vi "Circle detection.vi"() -> ()   [LabVIEW 2014]
uses:
  Resources/Global.vi
  <vilib>/vision/NI_Vision_Development_Module.lvlib
panel:
  in  "Circle Index":i32
  out "Number of Matches Returned":i32
  out "error out":errorcluster
  out "Image":T1(plugin-control)
  in  "milliseconds to wait":u32
  out "x-y":u32=19
  # "Do NOT un this VI. Instead run \"AR.Drone MAIN.vi\" and select the name of this VI in the dop-down menu at the Steup tab"
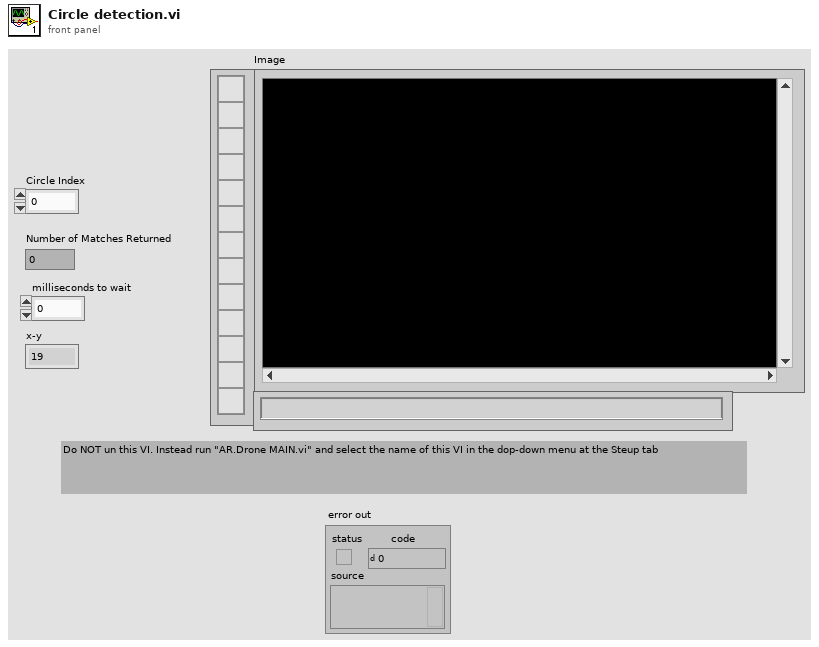
[diagram p1: front panel]
types:
  T1 = typedef "IMAQ Image.ctl" = refnum<image>
  T2 = typedef "Image Type" = u32
  T3 = cluster{"Position":cluster{"X":sgl, "Y":sgl}, "Radius":dbl, "Score":dbl}[]
  T4 = cluster{"Position":cluster{"X":sgl, "Y":sgl}, "Radius":dbl, "Score":dbl}
  T5 = cluster{"Left":i32, "Top":i32, "Right":i32, "Bottom":i32}
  T6 = typedef "Control cluster.ctl" = cluster{"Roll":sgl, "Pitch":sgl, "Vertical Speed":sgl, "Yaw Speed":sgl}
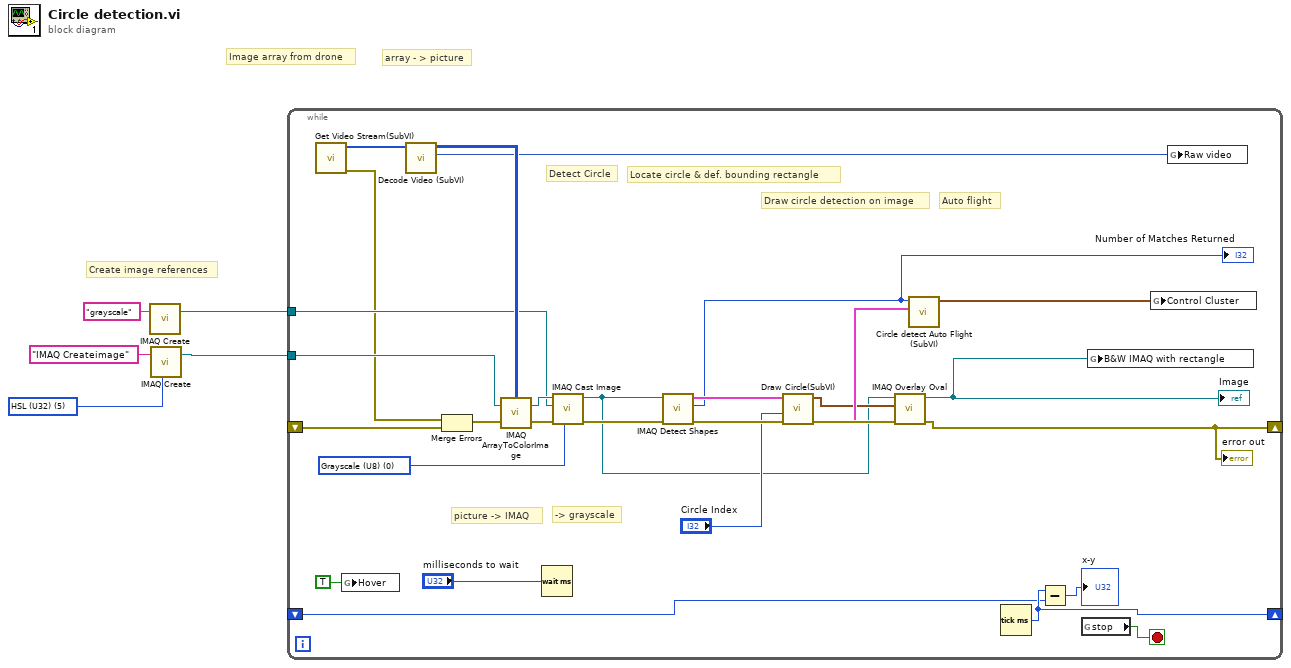
[diagram p0: block diagram]
diagram:
  w3 = T2 5 items=["Grayscale (U8)", "Grayscale (I16)", "Grayscale (SGL)", "Complex (CSG)", "RGB (U32)", "HSL (U32)", "RGB (U64)", "Grayscale (U16)"] ("Image Type")
  # "Create image references"
  # "array - > picture"
  # "Image array from drone"
  n1 = call "IMAQ Create"("Image Name"="grayscale") -> ("New Image"=w2:T1)  [unwired: 4 in, 1 out]
  n2 = call "IMAQ Create"("Image Name"="IMAQ Createimage", "Image Type"=w3) -> ("New Image"=w4:T1)  [unwired: 3 in, 1 out]
  n3 = while {
    shift-right: [w30] -> _
    shift-left: _ -> [w29]
    shift-right: [w6] -> _
    shift-left: _ -> [w10]
    tunnel: w4 -> [w14]
    tunnel: w2 -> [w13]
    stop <- w16 stop-if-true
    w25 = T2 0 items=["Grayscale (U8)", "Grayscale (I16)", "Grayscale (SGL)", "Complex (CSG)", "RGB (U32)", "HSL (U32)", "RGB (U64)", "Grayscale (U16)"] ("Image Type")
    # "-> grayscale"
    # "picture -> IMAQ"
    # "Auto flight"
    # "Draw circle detection on image"
    # "Locate circle & def. bounding rectangle"
    # "Detect Circle"
    n4 = call "Get Video Stream(SubVI).vi"() -> ("error out"=w11:errorcluster, "ImgData"=w32:u8[])  [unwired: 10 in]
    n5 = global write "Global.vi" "Hover"(TRUE) -> ()
    n6 = call "Decode Video (SubVI).vi"("ImgData"=w32) -> ("new picture"=w27:picture, "Array"=w31:u32[][])  [unwired: 9 in]
    n7 = Merge Errors(w11, w10) -> (w12:errorcluster)
    n8 = call "IMAQ ArrayToColorImage"("Image Pixels (U32)"=w31, "Image"=w14, "error in (no error)"=w12) -> ("Image Out"=w26:T1, "error out"=w15:errorcluster)  [unwired: 2 in]
    n9 = Wait (ms)(milliseconds to wait="milliseconds to wait") -> ()  [unwired: 1 out]
    n10 = call "IMAQ Cast Image"("Image Type"=w25, "error in (no error)"=w15, "Image Dst"=w13, "Image Src"=w26) -> ("error out"=w24:errorcluster, "Image Dst Out"=w8:T1)  [unwired: 6 in]
    n11 = call-poly "IMAQ Detect Shapes"("error in (no error)"=w24, "Image"=w8) -> ("error out"=w23:errorcluster, "Number of Matches Returned"=w7:i32, "Circles"=w22:T3)  [unwired: 7 in]
    "Number of Matches Returned" <- w7
    n12 = call "Draw Circle(SubVI).vi"("Circle Index"="Circle Index", "Circles"=w22) -> ("element"=w21:T4, "Bounding Rectangle out"=w9:T5)  [unwired: 7 in, 1 out]
    n13 = call "IMAQ Overlay Oval"("error in (no error)"=w23, "Bounding Rectangle"=w9, "Image"=w8) -> ("error out"=w6:errorcluster, "Image Out"=w19:T1)  [unwired: 7 in]
    "Image" <- w19
    "error out" <- w6
    n14 = call "Circle detect Auto Flight (SubVI).vi"("element"=w21, "Number of Matches Returned"=w7) -> ("Control Cluster out"=w20:T6)  [unwired: 9 in]
    n15 = Tick Count (ms)() -> (millisecond timer value=w30:u32)
    n16 = Subtract(x=w30, y=w29) -> (x-y=→"x-y":u32)
    n17 = global read "Global.vi" "stop"() -> (w16:bool)
    n18 = global write "Global.vi" "B&W IMAQ with rectangle"(w19) -> ()
    n19 = global write "Global.vi" "Control Cluster"(w20) -> ()
    n20 = global write "Global.vi" "Raw video"(w27) -> ()
  }
